vi "iSpy_Client.vi"() -> ()   [LabVIEW 2022 SP3]
panel:
  in  "stop":bool
  in  "Saving Files":path
  in  "Path":path
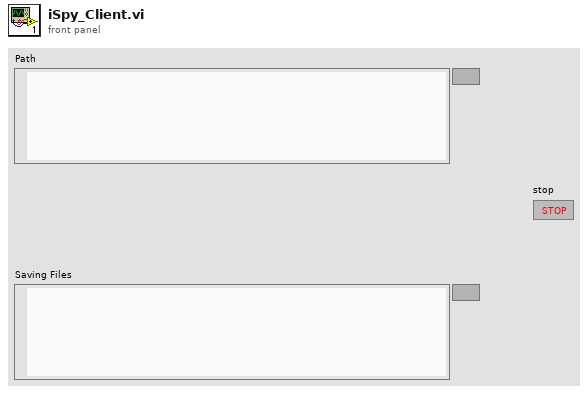
[diagram p1: front panel]
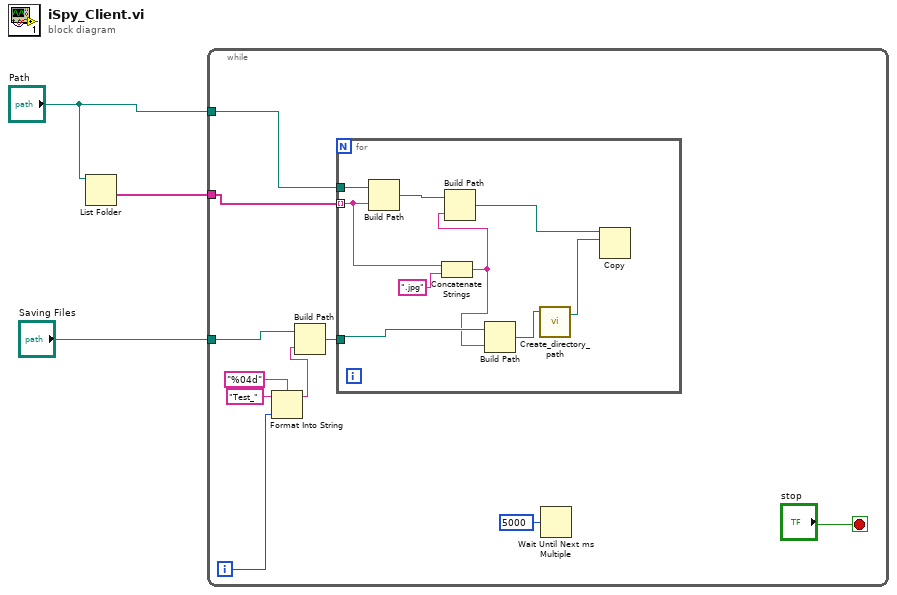
[diagram p0: block diagram]
diagram:
  n1 = List Folder(path="Path") -> (folder names=w1:string[])  [unwired: 3 in, 3 out]
  n2 = while {
    tunnel: "Path" -> [w13]
    tunnel: "Saving Files" -> [w12]
    tunnel: w1 -> [w4]
    i -> [w11]
    stop <- "stop" stop-if-true
    n3 = Format Into String(format string="%04d", initial string="Test_", w11) -> (resulting string=w9:string)  [unwired: 1 in, 1 out]
    n4 = Build Path(base path=w12, name or relative path=w9) -> (appended path=w7:path)
    n5 = for {
      tunnel: w13 -> [w22]
      tunnel: w4 -> [w17] mode=indexing
      tunnel: w7 -> [w21]
      n6 = Build Path(base path=w22, name or relative path=w17) -> (appended path=w18:path)
      n7 = Concatenate Strings(w17, ".jpg" ("string")) -> (w14:string)
      n8 = Build Path(base path=w18, name or relative path=w14) -> (appended path=w15:path)
      n9 = Build Path(base path=w21, name or relative path=w14) -> (appended path=w20:path)
      n10 = call "Create_directory_path.vi"("Path name"=w20) -> ("Path name Out"=w19:path)  [unwired: 2 in, 1 out]
      n11 = Copy(10:w19, 11:w15) -> ()  [unwired: 3 in, 3 out]
    }
    n12 = Wait Until Next ms Multiple(millisecond multiple=u32 5000) -> ()  [unwired: 1 out]
  }
